vi "FTDI - Read Channel.vi"(6 "index":i32, 8 "error in":errorcluster, 11 "Result":u8[](array[numeric])=[2, 14, 34, 1, 0, 66, 62, 41, 121, 0, 0, 0, 0, 1]) -> (0 "error out":errorcluster, 2 "Data Channel":T1, 3 "Success":bool, 5 "Prev Data?":bool)   [LabVIEW 2019]
uses:
  Controls/Global - Channel.vi
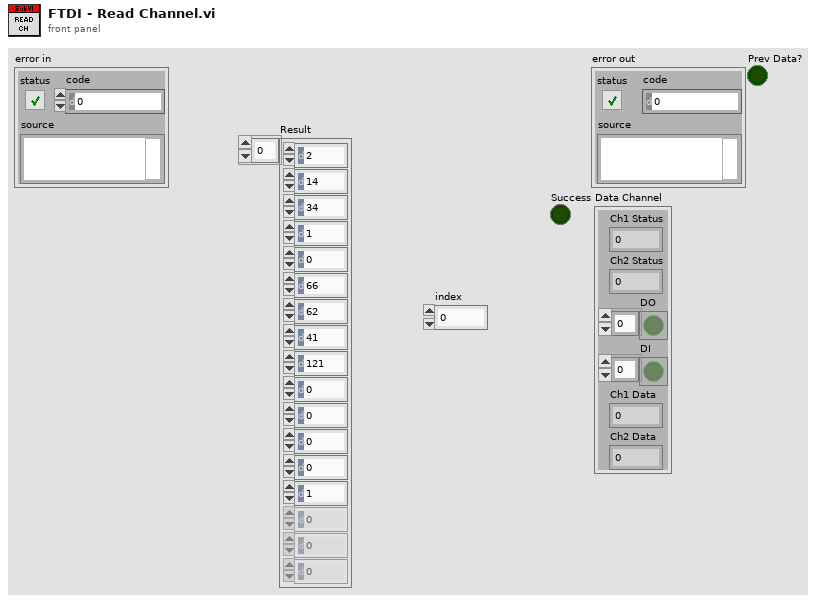
[diagram p1: front panel]
types:
  T1 = cluster{"Ch1 Status":u8, "Ch2 Status":u8, "DO":bool[], "DI":bool[], "Ch1 Data":sgl, "Ch2 Data":sgl}
  T2 = typedef "UDP - Event.ctl" = u16
  T3 = typedef "UDP - Status.ctl" = u16
  T4 = cluster{"Channels":cluster{"Ch1":sgl, "Ch2":sgl, "Ch3":sgl, "Ch4":sgl, "Ch5":sgl, "Ch6":sgl, "Ch7":sgl, "Ch8":sgl, "Ch9":sgl, "Ch10":sgl, "Ch11":sgl, "Ch12":sgl, "Ch13":sgl, "Ch14":sgl, "Ch15":sgl, "Ch16":sgl}, "Event":T2, "Status":T3, "IP":string}[]
  T5 = cluster{"Channels":cluster{"Ch1":sgl, "Ch2":sgl, "Ch3":sgl, "Ch4":sgl, "Ch5":sgl, "Ch6":sgl, "Ch7":sgl, "Ch8":sgl, "Ch9":sgl, "Ch10":sgl, "Ch11":sgl, "Ch12":sgl, "Ch13":sgl, "Ch14":sgl, "Ch15":sgl, "Ch16":sgl}, "Event":T2, "Status":T3, "IP":string}
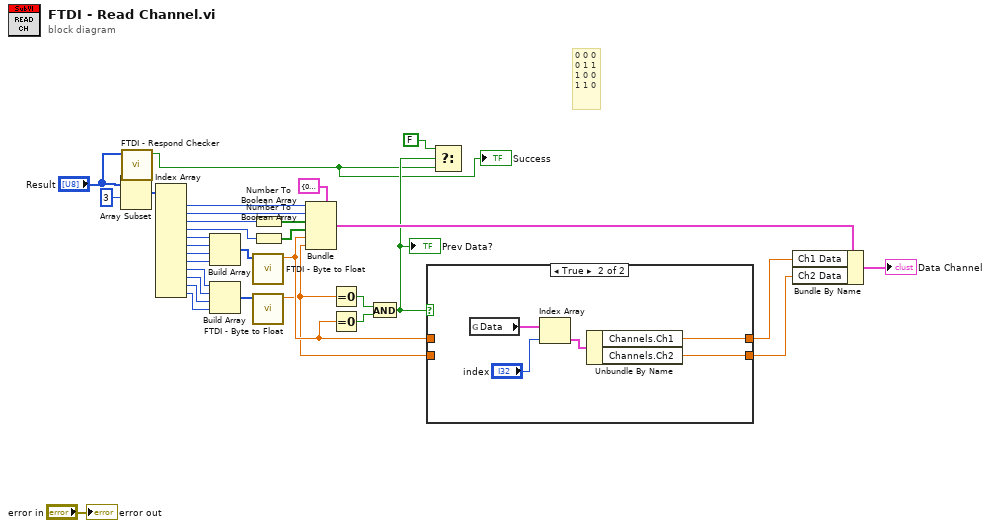
[diagram p0: block diagram]
diagram:
  # "0 0 0\n0 1 1\n1 0 0\n1 1 0"
  n1 = Array Subset(array="Result", index=3) -> (w31:u8[])  [unwired: 1 in]
  n2 = call "FTDI - Respond Checker.vi"("Read Data"="Result") -> ("Success"=w1:bool)  [unwired: 10 in]
  "Success" <- w1
  n3 = Index Array(array=w31) -> (element #1=w18:u8, element #2=w17:u8, element #3=w16:u8, element #4=w15:u8, element #5=w26:u8, element #6=w25:u8, element #7=w24:u8, element #8=w23:u8, element #9=w22:u8, element #10=w21:u8, element #11=w20:u8, element #12=w19:u8)  [unwired: 12 in]
  n4 = Build Array(w26, w25, w24, w23) -> (w30:u8[])
  n5 = Build Array(w22, w21, w20, w19) -> (w29:u8[])
  n6 = call "FTDI - Byte to Float.vi"("Byte"=w30) -> ("Float"=w11:sgl)  [unwired: 10 in]
  n7 = call "FTDI - Byte to Float.vi"("Byte"=w29) -> ("Float"=w10:sgl)  [unwired: 10 in]
  n8 = Number To Boolean Array(number=w16) -> (Boolean array=w14:bool[])
  n9 = Number To Boolean Array(number=w15) -> (Boolean array=w13:bool[])
  n10 = Bundle(cluster=T1 {"Ch1 Status"=0, "Ch2 Status"=0, "DO"=[], "DI"=[], "Ch1 Data"=0.0, "Ch2 Data"=0.0} ("output cluster"), "Ch1 Status"=w18, "Ch2 Status"=w17, "DO"=w14, "DI"=w13, "Ch1 Data"=w11, "Ch2 Data"=w10) -> (w7:T1)
  n11 = Equal To 0?(x=w10) -> (x = 0?=w9:bool)
  n12 = Equal To 0?(x=w11) -> (x = 0?=w8:bool)
  n13 = And(x=w9, y=w8) -> (x .and. y?=w3:bool)
  "Prev Data?" <- w3
  n14 = case shown="True" w3 {
    tunnel: w11 -> [w34 _]
    tunnel: w10 -> [w33 _]
    tunnel: [w34 w36] -> w5
    tunnel: [w33 w35] -> w4
    frame False {
    }
    frame True {
      n15 = global read "Global - Channel.vi" "Data"() -> (w37:T4)
      n16 = Index Array(array=w37, index="index") -> (element=w39:T5)
      n17 = Unbundle By Name(w39) -> ("Channels.Ch1"=w36:sgl, "Channels.Ch2"=w35:sgl)
    }
  }
  n18 = Select(t=FALSE, s=w3, f=w1) -> ()  [unwired: 1 out]
  n19 = Bundle By Name(cluster=w7, "Ch1 Data"=w5, "Ch2 Data"=w4) -> (→"Data Channel":T1)
  "error out" <- "error in"
